vi "Build a Filter Bank Tree.vi"() -> ()   [LabVIEW 2023]
doc: "A filter bank tree is a type of non-uniform filter bank. This example demonstrates how to build a 3-level filter bank tree. Each level contains a 2-band perfect reconstruction filter bank. You also can append M-band perfect reconstruction filter banks to the filter bank tree. The filter bank tree reconstructs signals perfectly as long as the appended filter banks are perfect reconstruction filter banks.\n\nComplete the following steps to use this example.\n1) Run this VI.\n2) Select the <b>Tree Structure (Analysis Bank)</b>. Observe the corresponding structure of the synthesis bank.\n3) Set the <b>Subband Index</b> to examine the magnitude response of each subband filter or filter bank."
uses:
  <vilib>/addons/Digital Filter Design/NI_DigFilter_FilterBank.lvlib
panel:
  in  "stop":bool
  in  "Subband Index":T1(ring)
  out "Tree Structure (Synthesis Bank)":u16(ring)
  in  "Tree Structure (Analysis Bank)":u16(ring)
  out "Magnitude Responses":cluster{"Y":dbl[], "Y":dbl[]}[](graph)
  # "Select Help>>Show Context Help and move the cursor over the VI icon for more information."
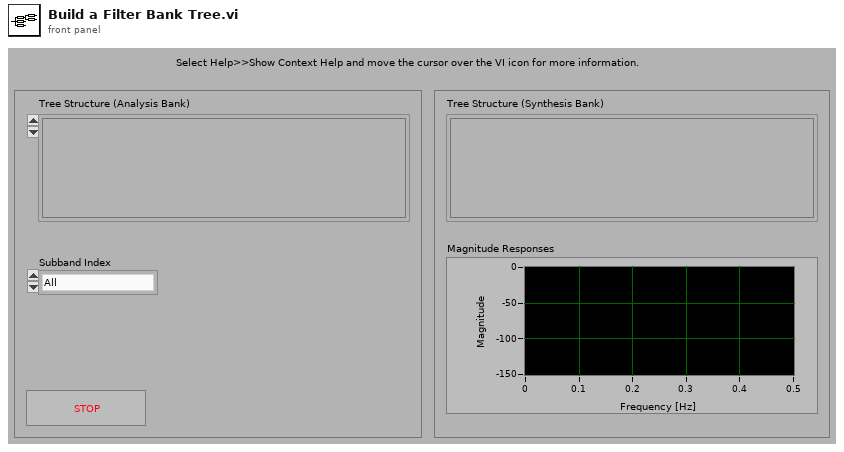
[diagram p1: front panel]
types:
  T1 = enum16{"All", "Subband 0", "Subband 1", "Subband 2", "Subband 3"}
  T2 = typedef "NI_DigFilter_FilterBank.lvlib/DFD Filter Bank Obj.ctl" = cluster{"mFBank_AnalysisFilters":T3[], "mFBank_SynthesisFilters":T3[], "mFBank_#Bands":i32, "mFBank_ProcMethod":T8, "mFBank_Coeffs":dbl[], "mFBank_Gain":dbl, "mFBank_Delay":i32, "mFBank_Type":T9}
  T3 = typedef "NI_DigFilterLicensed.lvlib/DFD Multirate Filter Obj.ctl" = cluster{"mMRate_Structure":enum16{"CIC", "FIR", "IIR", "Lattice"}, "mMRate_Mode":T4, "mMRate_Factor":i32, "mMRate_FIRParams":cluster{"mMRate_FIR_H":dbl[], "mMRate_FIR_IsNyquist?":bool, "mMRate_FIR_IsSymmetric?":bool}, "mMRate_CICParams":cluster{"mMRate_CIC_#Stage":i32, "mMRate_CIC_Lag":i32, "mMRate_CIC_Type":enum16{"Lowpass", "Highpass"}}, "mMRate_Order":i32, "mMRate_Version":string, "mMRate_Comments":string, "mMRate_RationalFactor":cluster{"mMRate_L":i32, "mMRate_M":i32}, "mMRate_Fs":dbl, "mMRate_Quantized?":bool, "mMRate_QFilterGain":dbl, "mMRate_CoefWl":i16, "mMRate_Scaling":cluster{"mMRate_ScaleByPowerOf2?":bool, "mMRate_ScaleType":T5}, "mMRate_InputWl":i16, "mMRate_OutputWl":i16, "mMRate_OutputMode":T6, "mMRate_MultMode":T7, "mMRate_BitPruning":bool, "mMRate_GainWl":i16, "mMRate_OutputFwl":i16, "mMRate_SumIwl":i16, "mMRate_InputIwl ":i16, "mMRate_SumWl":i16, "mMRate_CoefIwl":i16}
  T4 = typedef "NI_DigFilterLicensed.lvlib/DFD Multirate Mode.ctl" = i16
  T5 = typedef "NI_DigFilterLicensed.lvlib/DFD Coef Norm Type.ctl" = enum16{"No Norm", "Time Domain 1-Norm", "Time Domain 2-Norm", "Time Domain Inf-Norm"}
  T6 = typedef "NI_DigFilterLicensed.lvlib/DFD Round-off Mode.ctl" = enum16{"Nearest", "Truncation"}
  T7 = typedef "NI_DigFilterLicensed.lvlib/DFD FXP MRate Multiply Mode.ctl" = enum16{"Truncated", "Full"}
  T8 = typedef "NI_DigFilter_FilterBank.lvlib/DFD Filter Bank Processing Method.ctl" = enum16{"General", "2-Band QMF Lattice", "Cosine-Modulated"}
  T9 = typedef "NI_DigFilter_FilterBank.lvlib/DFD Filter Bank Type.ctl" = u16
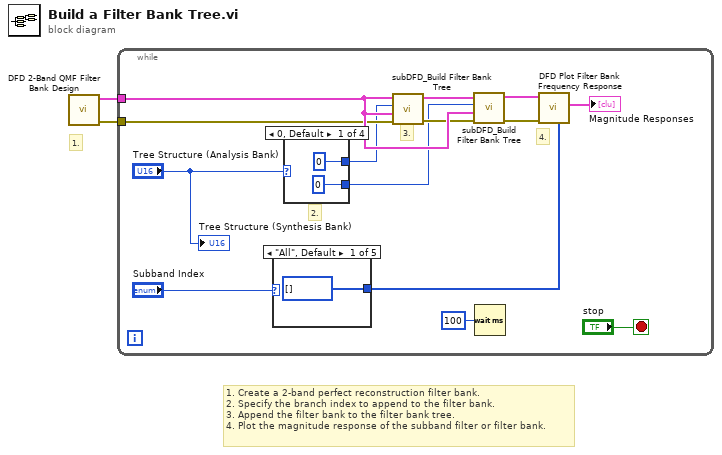
[diagram p0: block diagram]
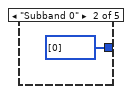
[diagram p2: hidden frame]
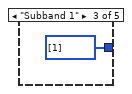
[diagram p3: hidden frame]
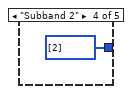
[diagram p4: hidden frame]
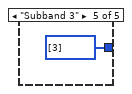
[diagram p5: hidden frame]
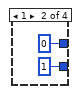
[diagram p6: hidden frame]
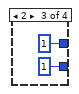
[diagram p7: hidden frame]
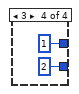
[diagram p8: hidden frame]
diagram:
  # "1. Create a 2-band perfect reconstruction filter bank.\n2. Specify the branch index to append to the filter bank.\n3. Append the filter bank to the filter bank tree.\n4. Plot the magnitude response of the subband filter or filter bank."
  # "1."
  n1 = call <vilib>:"DFD 2-Band QMF Filter Bank Design.vi"() -> ("error out"=w1:errorcluster, "filter bank out"=w2:T2)  [unwired: 9 in, 1 out]
  n2 = while {
    tunnel: w2 -> [w16]
    tunnel: w1 -> [w13]
    stop <- "stop" stop-if-true
    # "4."
    # "2."
    # "3."
    n3 = case shown="\"All\", Default" "Subband Index" {
      tunnel: [i32[] [] ("subband index") i32[] [0] ("subband index") i32[] [1] ("subband index") i32[] [2] ("subband index") i32[] [3] ("subband index")] -> w5
      frame "All", Default {
      }
      frame "Subband 0" {
      }
      frame "Subband 1" {
      }
      frame "Subband 2" {
      }
      frame "Subband 3" {
      }
    }
    n4 = case shown="0, Default" "Tree Structure (Analysis Bank)" {
      tunnel: [0 ("branch index") 0 ("branch index") 1 ("branch index") 1 ("branch index")] -> w9
      tunnel: [0 ("branch index") 1 ("branch index") 1 ("branch index") 2 ("branch index")] -> w8
      frame 0, Default {
      }
      frame 1 {
      }
      frame 2 {
      }
      frame 3 {
      }
    }
    n5 = call "subDFD_Build Filter Bank Tree.vi"("error in (no error)"=w13, "bank to append"=w16, "branch index"=w9, "tree in"=w16) -> ("error out"=w15:errorcluster, "tree out"=w4:T2)  [unwired: 6 in]
    n6 = call "subDFD_Build Filter Bank Tree.vi"("error in (no error)"=w15, "bank to append"=w16, "branch index"=w8, "tree in"=w4) -> ("error out"=w14:errorcluster, "tree out"=w3:T2)  [unwired: 6 in]
    n7 = Wait (ms)(milliseconds to wait=u32 100) -> ()  [unwired: 1 out]
    n8 = call <vilib>:"DFD Plot Filter Bank Frequency Response.vi"("subband index"=w5, "error in (no error)"=w14, "filter bank in"=w3) -> ("magnitude responses"=→"Magnitude Responses":cluster{"Y":dbl[], "Y":dbl[]}[])  [unwired: 5 in, 3 out]
    "Tree Structure (Synthesis Bank)" <- "Tree Structure (Analysis Bank)"
  }
